vi "Reset.vi"(8 "error in (no error)":errorcluster, 11 "VISA resource name":refnum<visa-resource-name>) -> (0 "error out":errorcluster, 3 "VISA resource name out":refnum<visa-resource-name>)   [LabVIEW 2019, in "DS360.lvlib"]
uses:
  DS360.lvlib
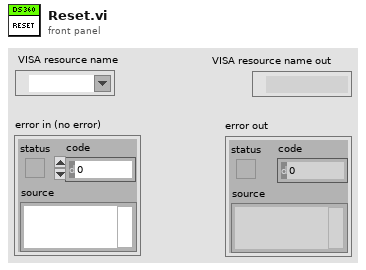
[diagram p1: front panel]
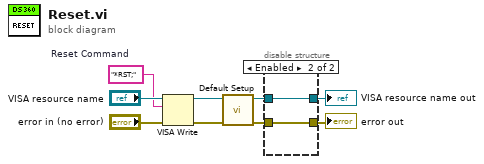
[diagram p0: block diagram]
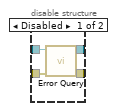
[diagram p2: hidden frame]
diagram:
  w7 = "*RST;"  # Reset Command
  n1 = VISA Write(VISA resource name="VISA resource name", write buffer=w7, error in (no error)="error in (no error)") -> (VISA resource name out=w5:refnum<visa-resource-name>, error out=w6:errorcluster)  [unwired: 1 out]
  n2 = call "Default Setup.vi"("error in (no error)"=w6, "VISA resource name"=w5) -> ("error out"=w4:errorcluster, "VISA resource name out"=w3:refnum<visa-resource-name>)  [unwired: 8 in]
  n3 = disable-structure shown="Enabled" {
    disable-tunnel: w4 -> [w13 w14]
    disable-tunnel: w3 -> [w12 w15]
    disable-tunnel: [w11 w15] -> w2
    disable-tunnel: [w10 w14] -> w1
    frame Disabled {
      n4 = call "Error Query.vi"("error in (no error)"=w13, "VISA resource name"=w12) -> ("error out"=w10:errorcluster, "VISA resource name out"=w11:refnum<visa-resource-name>)  [unwired: 6 in, 2 out]
    }
    frame Enabled {
    }
  }
  "error out" <- w1
  "VISA resource name out" <- w2
